vi "Enqueue N Items.vi"(7 "Add to Queue? (T)":bool=TRUE, 8 "Error In":errorcluster, 10 "Enqueue N":string[](array[string]), 11 "Queue Ref In":refnum<queue>) -> (0 "Error Out":errorcluster, 3 "Queue Ref Out":refnum<queue>)   [LabVIEW 2016, in "SLL QSM.lvlib"]
doc: "Add Multiple States to the Queue based on the input boolean flag - \"Add to Queue?\"."
uses:
  SLL QSM.lvlib
  Typedefs/Queue Type.ctl
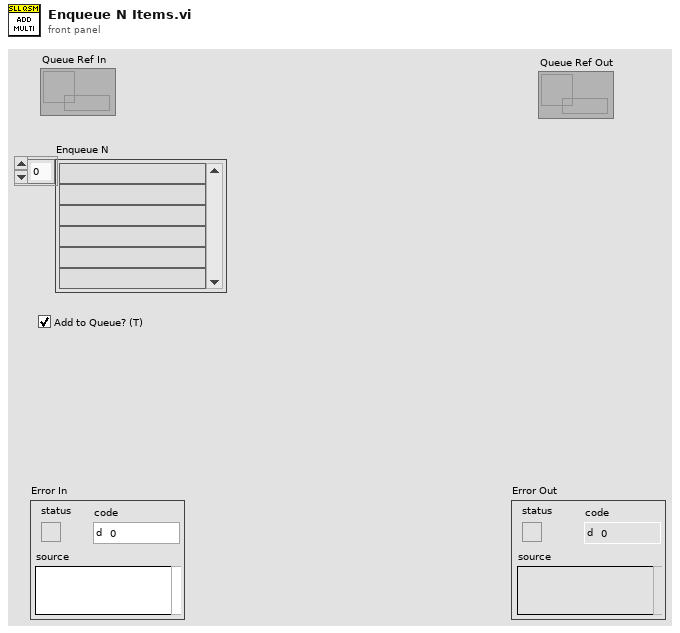
[diagram p1: front panel]
types:
  T1 = typedef "SLL QSM.lvlib/Queue Type.ctl" = cluster{"State":string, "Data":variant}
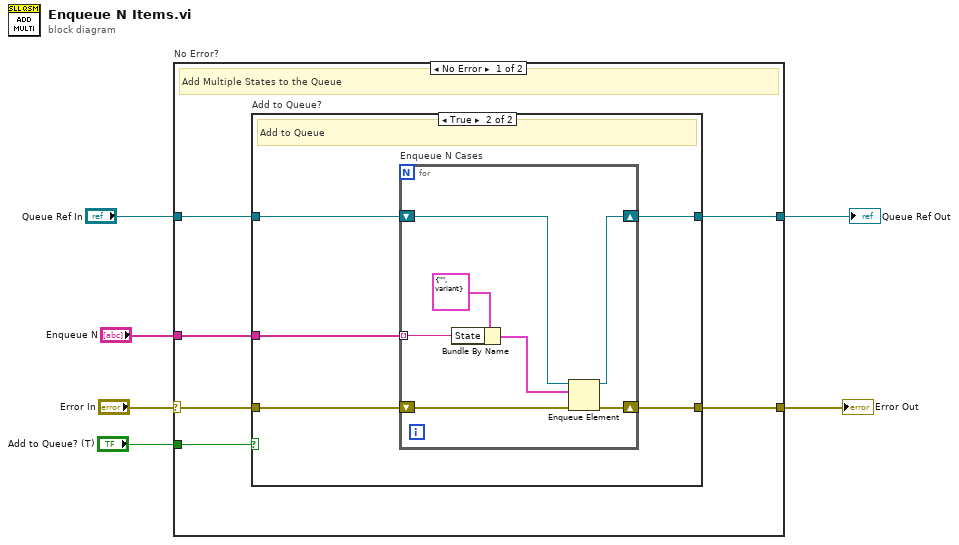
[diagram p0: block diagram]
diagram:
  n1 = case "No Error?" shown="No Error" "Error In" {
    selector: "Error In" -> [w10 w28]
    tunnel: [w12 w28] -> w6
    tunnel: "Enqueue N" -> [w11 _]
    tunnel: "Add to Queue? (T)" -> [w9 _]
    tunnel: "Queue Ref In" -> [w8 w27]
    tunnel: [w7 w27] -> w1
    frame No Error {
      # "Add Multiple States to the Queue"
      n2 = case "Add to Queue?" shown="True" w9 {
        tunnel: w10 -> [w14 w16]
        tunnel: [w14 w19] -> w12
        tunnel: w11 -> [_ w18]
        tunnel: w8 -> [w13 w17]
        tunnel: [w13 w15] -> w7
        frame False {
          # "Skip adding to the Queue"
        }
        frame True {
          # "Add to Queue"
          n3 = for "Enqueue N Cases" {
            shift-right: [w25] -> w19
            shift-left: w16 -> [w26]
            tunnel: w18 -> [w23] mode=indexing
            shift-right: [w20] -> w15
            shift-left: w17 -> [w21]
            n4 = Bundle By Name(cluster=T1 {"State"="", "Data"=variant} ("Queue Type"), "State"=w23) -> (w22:T1)
            n5 = Enqueue Element(queue=w21, element=w22, error in (no error)=w26) -> (queue out=w20:refnum<queue>, error out=w25:errorcluster)  [unwired: 1 in, 1 out]
          }
        }
      }
    }
    frame Error {
    }
  }
  "Error Out" <- w6
  "Queue Ref Out" <- w1
